vi "CheckHandle.vi"(8 "Error In":errorcluster, 10 "Resource In":T1, 11 "Handle In":string) -> (0 "Error Out":errorcluster, 1 "VISA Resource":refnum<visa-resource-name>, 2 "Handle Connected?":bool, 3 "Handle Out":string)   [LabVIEW 2018, in "AcPwrPlugins.lvlib" / "NHRGridSim.lvclass"]
doc: "This VI checks that the instrument name is valid."
uses:
  NHRGridSim.lvclass
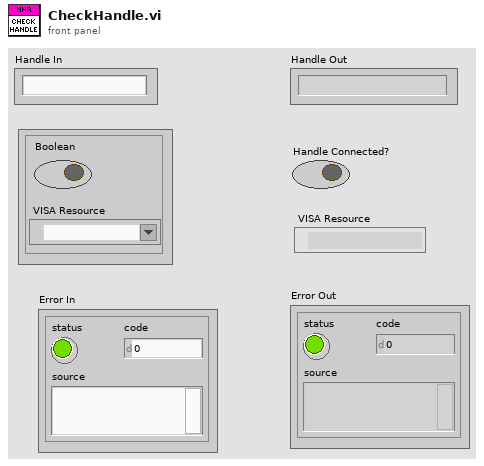
[diagram p1: front panel]
types:
  T1 = cluster{"Boolean":bool, "VISA Resource":refnum<visa-resource-name>}
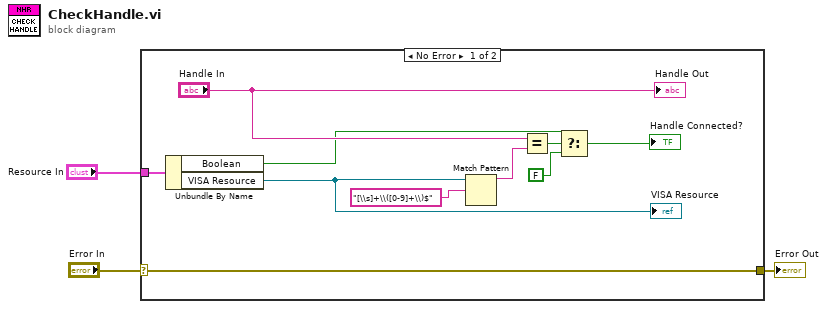
[diagram p0: block diagram]
diagram:
  n1 = case shown="No Error" "Error In" {
    selector: "Error In" -> [w12 w14]
    tunnel: [w12 w14] -> w2
    tunnel: "Resource In" -> [w4 _]
    frame No Error {
      n2 = Unbundle By Name(w4) -> ("Boolean"=w5:bool, "VISA Resource"=w10:refnum<visa-resource-name>)
      "VISA Resource" <- w10
      n3 = Match Pattern(string=w10, regular expression="[\\s]+\\([0-9]+\\)$") -> (before substring=w7:string)  [unwired: 1 in, 3 out]
      n4 = Equal?(x="Handle In", y=w7) -> (x = y?=w9:bool)
      n5 = Select(t=w5, s=w9, f=FALSE) -> (s? t:f=→"Handle Connected?":bool)
      "Handle Out" <- "Handle In"
    }
    frame Error {
    }
  }
  "Error Out" <- w2
